vi "TX Message.vi"(8 "error in (no error)":errorcluster, 10 "variant":variant, 11 "Engine RPM in":refnum<class "Supported PIDs.lvclass">) -> (0 "error out":errorcluster, 3 "Engine RPM out":refnum<class "Supported PIDs.lvclass">)   [LabVIEW 2011, in "Supported PIDs.lvclass"]
uses:
  Supported PIDs.lvclass
  PID.lvclass
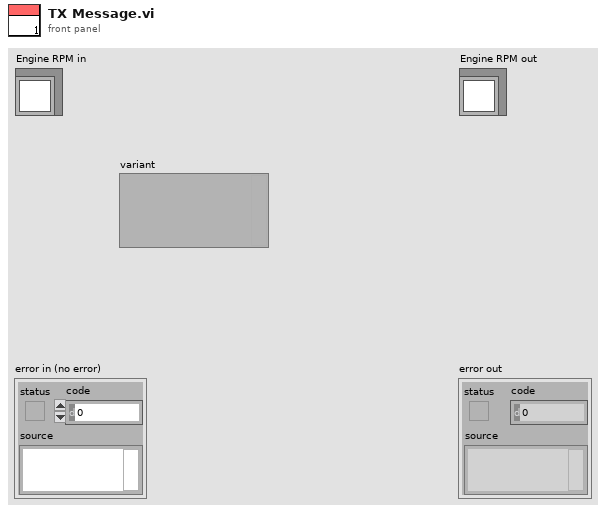
[diagram p1: front panel]
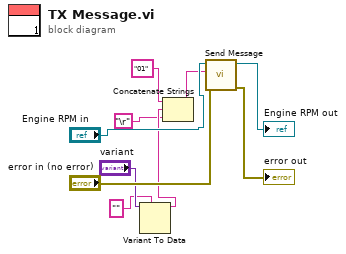
[diagram p0: block diagram]
diagram:
  n1 = Variant To Data(type="" ("TX Message"), Variant="variant") -> (data=w2:string)  [unwired: 1 in, 1 out]
  n2 = Concatenate Strings("01" ("TX Message"), w2, "\r") -> (w3:string)
  n3 = call "Send Message.vi"("error in (no error)"="error in (no error)", "TX Message"=w3, "PID in"="Engine RPM in") -> ("error out"=→"error out":errorcluster, "PID out"=→"Engine RPM out":refnum<class "Supported PIDs.lvclass">)  [unwired: 7 in]
